vi "Inpterpolate4.vi"(0 "X":fxp<+/-,16,14>, 11 "input valid":bool=TRUE) -> (4 "X(t)":fxp<+/-,16,14>, 6 "X(t -1)":fxp<+/-,16,14>, 8 "X(t -2)":fxp<+/-,16,14>, 10 "X(t -3)":fxp<+/-,16,14>, 15 "output valid":bool)   [LabVIEW 2013]
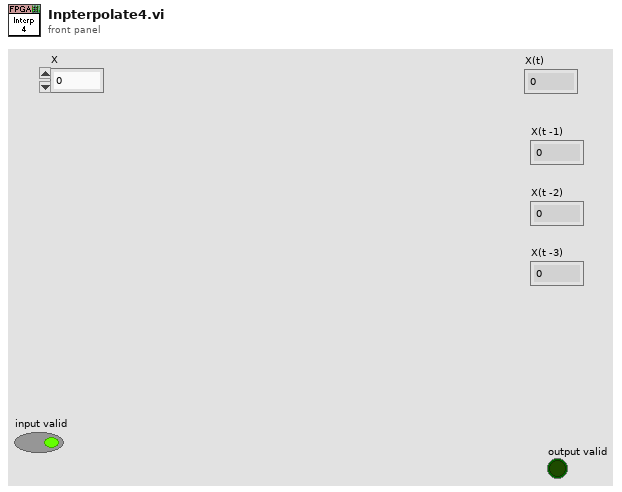
[diagram p1: front panel]
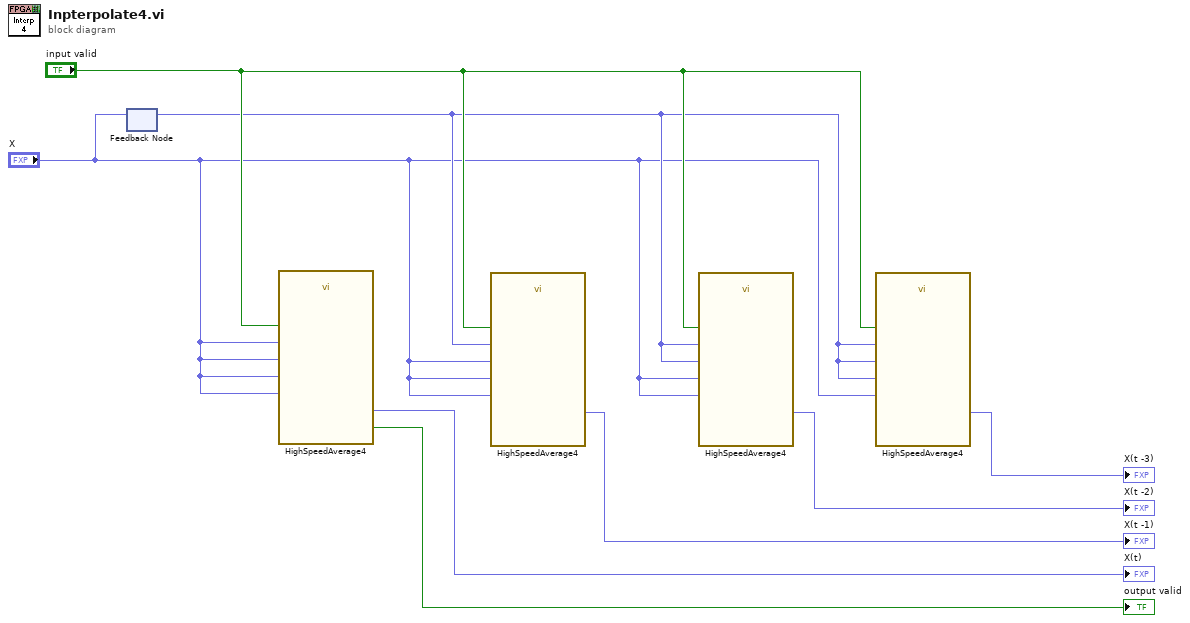
[diagram p0: block diagram]
diagram:
  n1 = feedback #1() -> (w2:fxp<+/-,16,14>)  [unwired: 1 in]
  n2 = feedback-in #1("X") -> ()
  n3 = call "HighSpeedAverage4.vi"("x 1"="X", "x 2"="X", "x 3"="X", "x 4"="X", "input valid"="input valid") -> ("average"=→"X(t)":fxp<+/-,16,14>, "output valid"=→"output valid":bool)  [unwired: 9 in]
  n4 = call "HighSpeedAverage4.vi"("x 1"=w2, "x 2"="X", "x 3"="X", "x 4"="X", "input valid"="input valid") -> ("average"=→"X(t -1)":fxp<+/-,16,14>)  [unwired: 9 in, 1 out]
  n5 = call "HighSpeedAverage4.vi"("x 1"=w2, "x 2"=w2, "x 3"="X", "x 4"="X", "input valid"="input valid") -> ("average"=→"X(t -2)":fxp<+/-,16,14>)  [unwired: 9 in, 1 out]
  n6 = call "HighSpeedAverage4.vi"("x 1"=w2, "x 2"=w2, "x 3"=w2, "x 4"="X", "input valid"="input valid") -> ("average"=→"X(t -3)":fxp<+/-,16,14>)  [unwired: 9 in, 1 out]
